vi "BusInOut_mode.vi"(8 "error in (no error)":errorcluster, 10 "Mode":string, 11 "BusInOut in":refnum<class "BusInOut.lvclass">) -> (0 "error out":errorcluster, 3 "BusInOut out":refnum<class "BusInOut.lvclass">)   [LabVIEW 2011, in "mbed_LVLibrary.lvlib" / "BusInOut.lvclass"]
uses:
  BusInOut.lvclass
  BusInOut.lvclass/BusInOut.ctl
  Transport Mechanisms/mbed/mbed.lvclass
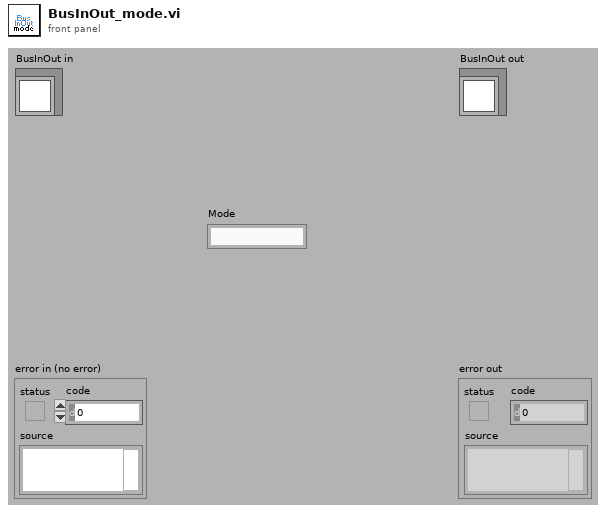
[diagram p1: front panel]
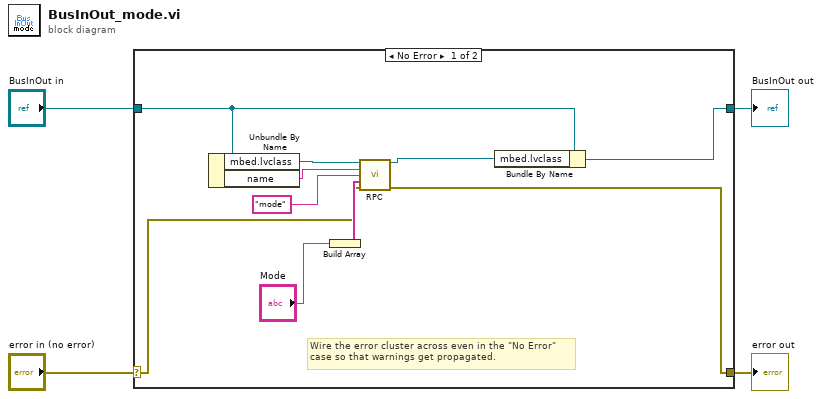
[diagram p0: block diagram]
diagram:
  n1 = case shown="No Error" "error in (no error)" {
    selector: "error in (no error)" -> [w7 w16]
    tunnel: [w6 w16] -> w3
    tunnel: [w13 w15] -> w1
    tunnel: "BusInOut in" -> [w14 w15]
    frame No Error {
      # "Wire the error cluster across even in the \"No Error\"\ncase so that warnings get propagated."
      n2 = Unbundle By Name(w14) -> ("mbed.lvclass"=w12:refnum<class "mbed.lvclass">, "name"=w11:string)
      n3 = Build Array("Mode") -> (w8:string[])
      n4 = call-dynamic "RPC.vi"("mbed in"=w12, "Name"=w11, "method"="mode", "Args"=w8, "error in (no error)"=w7) -> ("mbed out"=w9:refnum<class "mbed.lvclass">, "error out"=w6:errorcluster)  [unwired: 8 in, 1 out]
      n5 = Bundle By Name(cluster=w14, "mbed.lvclass"=w9) -> (w13:refnum<class "BusInOut.lvclass">)
    }
    frame Error {
    }
  }
  "error out" <- w3
  "BusInOut out" <- w1
